vi "Read Sorting Column.vi"(8 "error in":errorcluster, 11 "EngineTags in":refnum<class "EngineTags.lvclass">) -> (0 "error out":errorcluster, 2 "Sorting Column":i32, 3 "EngineTags out":refnum<class "EngineTags.lvclass">)   [LabVIEW 2013, in "PL Framework Configuration Tool.lvlib" / "EngineTags.lvclass"]
uses:
  EngineTags.lvclass
  EngineTags.lvclass/EngineTags.ctl
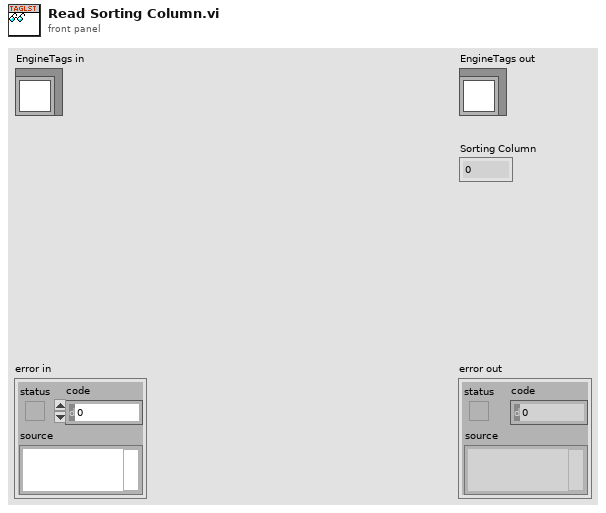
[diagram p1: front panel]
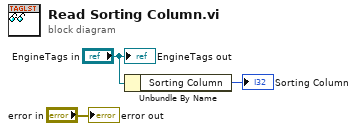
[diagram p0: block diagram]
diagram:
  n1 = Unbundle By Name("EngineTags in") -> ("Sorting Column"=→"Sorting Column":i32)
  "error out" <- "error in"
  "EngineTags out" <- "EngineTags in"
